vi "Start AsyncRepeatSum.vi"(8 "error in (no error)":errorcluster, 10 "B":i32, 11 "A":i32) -> (0 "error out":errorcluster, 1 "AsyncSum Event Register":refnum<event-registration>, 2 "LVUserEvent CallBack Reference":refnum<user-event>, 3 "Handle":u64)   [LabVIEW 2016, in "DemoSkeleton.lvlib"]
uses:
  DemoSkeleton.lvlib
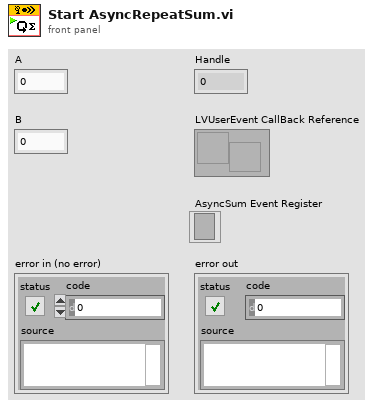
[diagram p1: front panel]
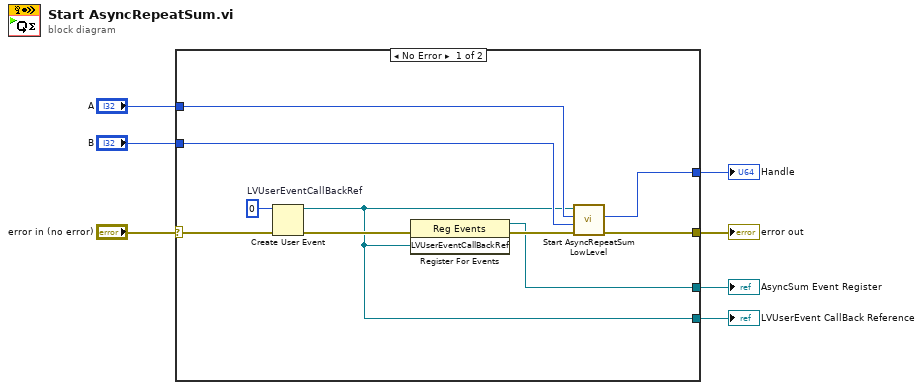
[diagram p0: block diagram]
diagram:
  n1 = case shown="No Error" "error in (no error)" {
    selector: "error in (no error)" -> [w12 w18]
    tunnel: [w9 _] -> w7
    tunnel: "A" -> [w16 _]
    tunnel: "B" -> [w15 _]
    tunnel: [w14 _] -> w4
    tunnel: [w13 w18] -> w3
    tunnel: [w8 _] -> w1
    frame No Error {
      w17 = i64 0  # LVUserEventCallBackRef
      n2 = Create User Event(user event datatype=w17, error in=w12) -> (user event=w9:refnum<user-event>, error out=w11:errorcluster)
      n3 = register-events(error in=w11, w9) -> (reference out=w8:refnum<event-registration>, error out=w10:errorcluster)  [unwired: 1 in]
      n4 = call "Start AsyncRepeatSum LowLevel.vi"("error in"=w10, "B"=w15, "A"=w16, "LVUserEventCallBackRef"=w9) -> ("error out"=w13:errorcluster, "Handle"=w14:u64)  [unwired: 6 in]
    }
    frame Error {
    }
  }
  "Handle" <- w4
  "error out" <- w3
  "LVUserEvent CallBack Reference" <- w7
  "AsyncSum Event Register" <- w1
